vi "QNET_ROTPEN_Pendulum_MOD.vi"(2 "offset (deg)":dbl=-180.0, 3 "mod angle (deg)":dbl=-180.0, 4 "gamma (deg)":dbl, 5 "gamma (rad)":dbl) -> (0 "gamma mod (deg)":dbl, 1 "gamma mod (rad)":dbl)   [LabVIEW 2021]
doc: "This VI calculates the modulus of the angle 'gamma' in degrees and radians and applies a given angular offset."
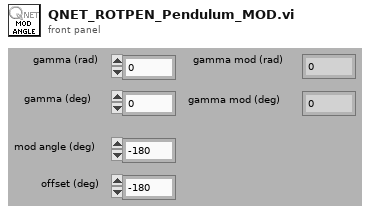
[diagram p1: front panel]
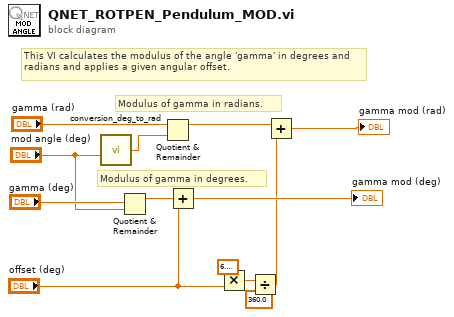
[diagram p0: block diagram]
diagram:
  # "This VI calculates the modulus of the angle 'gamma' in degrees and radians and applies a given angular offset."
  # "Modulus of gamma in degrees."
  # "Modulus of gamma in radians."
  n1 = call "conversion_deg_to_rad.vi"("Angle (deg)"="mod angle (deg)") -> ("Angle (rad)"=w1:dbl)
  n2 = Quotient & Remainder(x="gamma (deg)", y="mod angle (deg)") -> (x-y*floor(x/y)=w12:dbl)  [unwired: 1 out]
  n3 = Quotient & Remainder(x="gamma (rad)", y=w1) -> (x-y*floor(x/y)=w4:dbl)  [unwired: 1 out]
  n4 = Add(x=w12, y="offset (deg)") -> (x+y=→"gamma mod (deg)":dbl)
  n5 = Multiply(x=6.283185307179586, y="offset (deg)") -> (x*y=w8:dbl)
  n6 = Divide(x=w8, y=360.0) -> (x/y=w6:dbl)
  n7 = Add(x=w4, y=w6) -> (x+y=→"gamma mod (rad)":dbl)
